vi "Nikhil 3rd year.vi"() -> ()   [LabVIEW 2014]
panel:
  out "Boolean":bool
  out "Result 2":dbl
  out "Result":dynamicdata(graph)
  out "Filtered Signal 3":dynamicdata(graph) caption="Filtered Signal"
  out "Filtered Signal 2":dynamicdata(graph) caption="Filtered Signal"
  out "Filtered Signal":dynamicdata(graph)
  out "data 2":dbl
  out "data":dynamicdata(graph)
  in  "stop (F)":bool
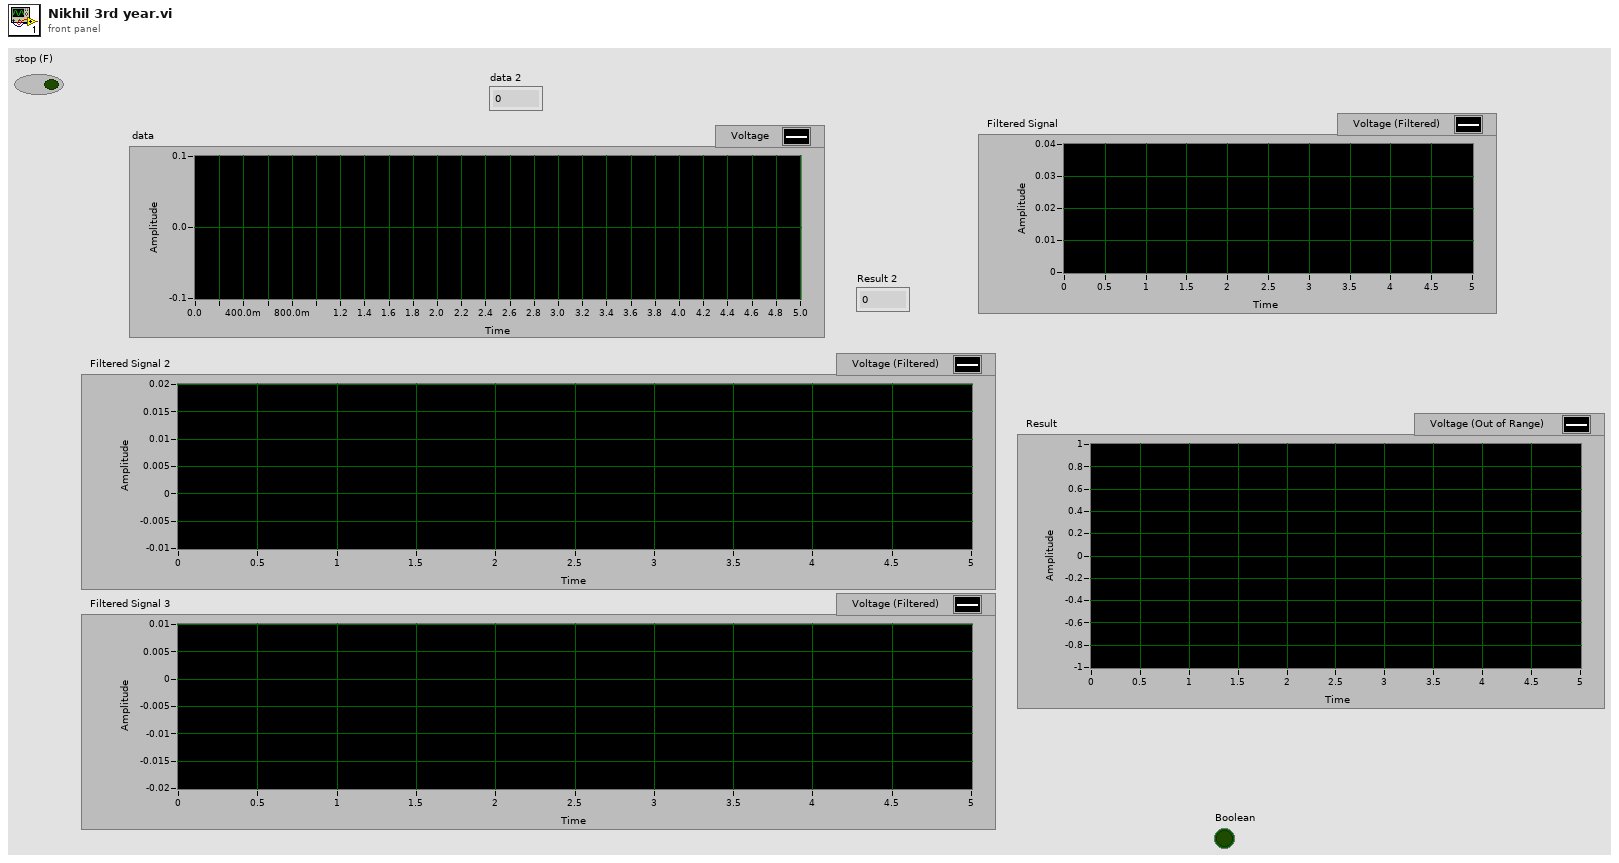
[diagram p1: front panel]
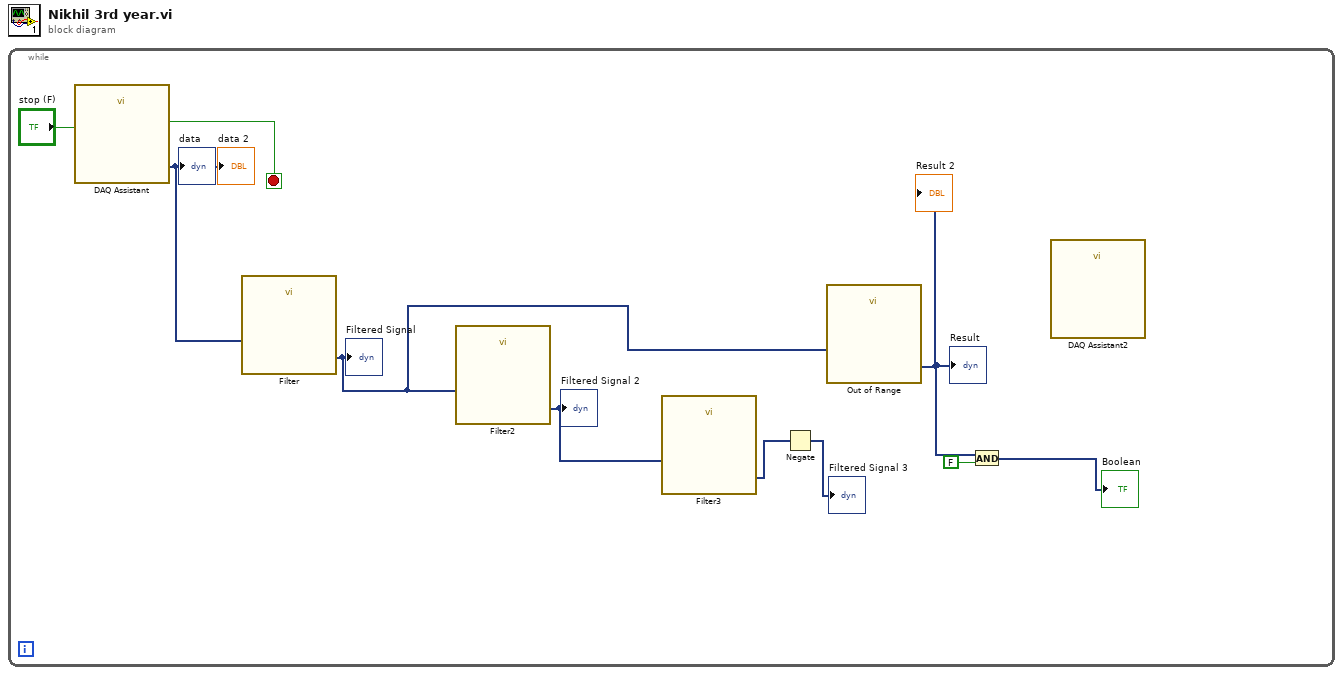
[diagram p0: block diagram]
diagram:
  n1 = while {
    stop <- w9 stop-if-true
    n2 = call "DAQ Assistant"("stop (F)"="stop (F)") -> ("data"=w8:dynamicdata, "stopped"=w9:bool)  [unwired: 15 in, 2 out]
    "data" <- w8
    "data 2" <- w8
    n3 = call "Filter"("Signal"=w8) -> ("Filtered Signal"=w2:dynamicdata)  [unwired: 9 in, 1 out]
    "Filtered Signal" <- w2
    n4 = call "Filter2"("Signal"=w2) -> ("Filtered Signal"=w7:dynamicdata)  [unwired: 9 in, 1 out]
    "Filtered Signal 2" <- w7
    n5 = call "Filter3"("Signal"=w7) -> ("Filtered Signal"=w6:dynamicdata)  [unwired: 9 in, 1 out]
    n6 = Negate(x=w6) -> (-x=→"Filtered Signal 3":dynamicdata)
    n7 = call "Out of Range"("Operand 1"=w2) -> ("Result"=w5:dynamicdata)  [unwired: 9 in, 1 out]
    "Result" <- w5
    "Result 2" <- w5
    n8 = And(x=w5, y=FALSE) -> (x .and. y?=→"Boolean":dynamicdata)
    n9 = call "DAQ Assistant2"() -> ()  [unwired: 17 in, 3 out]
  }
